vi "LOERN_GetTerms.vi"(0 "XRef":T12, 1 "State In":T10={"Inputs"=1, "SelectedIndex"=1, "ClassInfo"=[]}) -> (14 "Terms":T2, 15 "Fatal Error Out":T1)   [LabVIEW 2016, in "LV Object Event Registration Node.xnode"]
uses:
  LV Object Event Registration Node.xnode
  <vilib>/XNodeSupport/XNodeXNodeRef.ctl
  LOERN_State.ctl
  LOERN_ClassInfo.ctl
  <vilib>/XNodeSupport/XNodeTerm4Array.ctl
  <vilib>/XNodeSupport/XNodeTerm4.ctl
  <vilib>/XNodeSupport/XNodeString.ctl
  <vilib>/XNodeSupport/XNodeVariant.ctl
  <vilib>/XNodeSupport/XNodeRect32.ctl
  <vilib>/XNodeSupport/XNodeInt.ctl
  <vilib>/XNodeSupport/XNodeBool.ctl
  <vilib>/XNodeSupport/XNodeTermDirection.ctl
  <vilib>/XNodeSupport/XNodeErrorCluster.ctl
  <vilib>/XNodeSupport/NI_XNodeSupport.lvlib
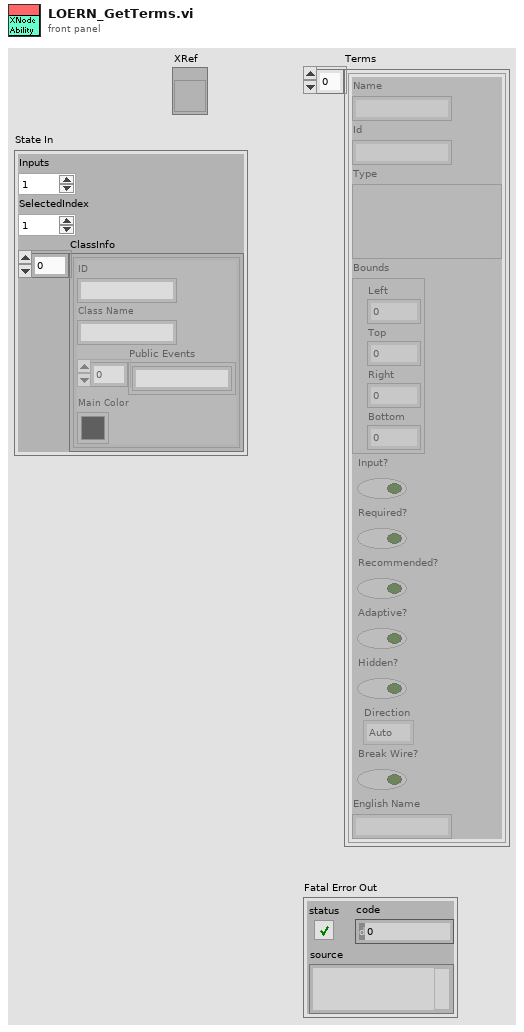
[diagram p1: front panel]
types:
  T1 = typedef "NI_XNodeSupport.lvlib/XNodeErrorCluster.ctl" = errorcluster
  T2 = typedef "NI_XNodeSupport.lvlib/XNodeTerm4Array.ctl" = T3[]
  T3 = typedef "NI_XNodeSupport.lvlib/XNodeTerm4.ctl" = cluster{"Name":T4, "Id":T4, "Type":T5, "Bounds":T6, "Input?":T8, "Required?":T8, "Recommended?":T8, "Adaptive?":T8, "Hidden?":T8, "Direction":T9, "Break Wire?":T8, "English Name":T4}
  T4 = typedef "NI_XNodeSupport.lvlib/XNodeString.ctl" = string
  T5 = typedef "NI_XNodeSupport.lvlib/XNodeVariant.ctl" = variant
  T6 = typedef "NI_XNodeSupport.lvlib/XNodeRect32.ctl" = cluster{"Left":T7, "Top":T7, "Right":T7, "Bottom":T7}
  T7 = typedef "NI_XNodeSupport.lvlib/XNodeInt.ctl" = i32
  T8 = typedef "NI_XNodeSupport.lvlib/XNodeBool.ctl" = bool
  T9 = typedef "NI_XNodeSupport.lvlib/XNodeTermDirection.ctl" = enum32{"Auto", "Up", "Down", "Left", "Right", "Center"}
  T10 = typedef "LV Object Event Registration Node.xnode/LOERN_State.ctl" = cluster{"Inputs":u16, "SelectedIndex":i16, "ClassInfo":T11[]}
  T11 = typedef "LV Object Event Registration Node.xnode/LOERN_ClassInfo.ctl" = cluster{"ID":string, "Class Name":string, "Public Events":string[], "Main Color":u32}
  T12 = typedef "NI_XNodeSupport.lvlib/XNodeXNodeRef.ctl" = refnum<vi>
  T13 = typedef "NI_XNodeSupport.lvlib/XNodeBounds.ctl" = cluster{"Width":T7, "Height":T7}
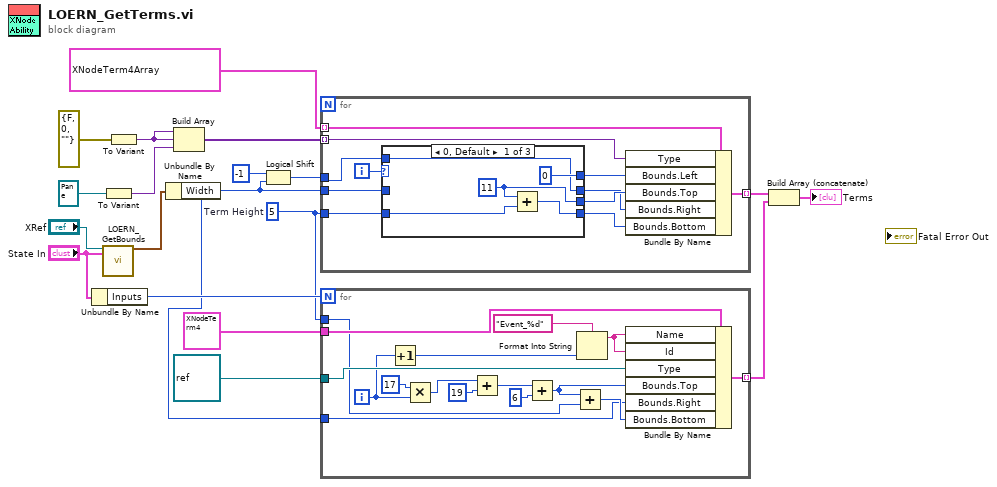
[diagram p0: block diagram]
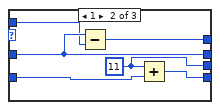
[diagram p2: hidden frame]
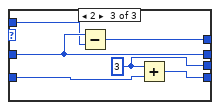
[diagram p3: hidden frame]
diagram:
  w4 = 5  # Term Height
  n1 = Unbundle By Name("State In") -> ("Inputs"=w10:u16)
  n2 = call "LOERN_GetBounds.vi"("XRef"="XRef", "State In"="State In") -> ("Bounds"=w12:T13)  [unwired: 16 in, 1 out]
  n3 = To Variant(anything=refnum<event-registration> refnum ("event registration refnum")) -> (Variant=w15:variant)
  n4 = To Variant(anything=errorcluster {"status"=FALSE, "code"=0, "source"=""} ("error in (no error)")) -> (Variant=w17:variant)
  n5 = Unbundle By Name(w12) -> ("Width"=w3:T7)
  n6 = Build Array(w17, w17, w15) -> (w14:variant[])
  n7 = Logical Shift(y=i16 -1, x=w3) -> (x << y=w1:T7)
  n8 = for {
    tunnel: T2 [{"Name"="Error_In", "Id"="error in", "Type"=variant, "Bounds"={"Left"=0, "Top"=0, "Right"=0, "Bottom"=0}, "Input?"=TRUE, "Required?"=FALSE, "Recommended?"=FALSE, "Adaptive?"=FALSE, "Hidden?"=FALSE, "Direction"=enum."Auto", "Break Wire?"=FALSE, "English Name"=""}, {"Name"="Error_Out", "Id"="error out", "Type"=variant, "Bounds"={"Left"=0, "Top"=0, "Right"=0, "Bottom"=0}, "Input?"=FALSE, "Required?"=FALSE, "Recommended?"=TRUE, "Adaptive?"=FALSE, "Hidden?"=FALSE, "Direction"=enum."Auto", "Break Wire?"=FALSE, "English Name"=""}, {"Name"="Obj_Event_Reg_Ref", "Id"="Object Event Registration Refnum", "Type"=variant, "Bounds"={"Left"=0, "Top"=0, "Right"=0, "Bottom"=0}, "Input?"=FALSE, "Required?"=FALSE, "Recommended?"=TRUE, "Adaptive?"=TRUE, "Hidden?"=FALSE, "Direction"=enum."Auto", "Break Wire?"=FALSE, "English Name"=""}] ("Terms") -> [w30] mode=indexing
    tunnel: w14 -> [w29] mode=indexing
    tunnel: [w28] -> w7 mode=indexing
    tunnel: w3 -> [w22]
    tunnel: w4 -> [w21]
    tunnel: w1 -> [w20]
    i -> [w27]
    n9 = case shown="0, Default" w27 {
      tunnel: [T7 0 ("Bounds.Left") w40 w46] -> w26
      tunnel: [w34 w39 w45] -> w25
      tunnel: [w31 w41 w47] -> w24
      tunnel: [w32 w37 w43] -> w23
      tunnel: w22 -> [_ w41 w47]
      tunnel: w21 -> [w33 w38 w44]
      tunnel: w20 -> [w31 w36 w42]
      frame 0, Default {
        w34 = T7 11 ("Bounds.Left")
        n10 = Add(x=w34, y=w33) -> (x+y=w32:T7)
      }
      frame 1 {
        w39 = T7 11 ("Bounds.Left")
        n11 = Subtract(x=w41, y=w36) -> (x-y=w40:T7)
        n12 = Add(x=w39, y=w38) -> (x+y=w37:T7)
      }
      frame 2 {
        w45 = T7 3 ("Bounds.Left")
        n13 = Subtract(x=w47, y=w42) -> (x-y=w46:T7)
        n14 = Add(x=w45, y=w44) -> (x+y=w43:T7)
      }
    }
    n15 = Bundle By Name(cluster=w30, "Type"=w29, "Bounds.Left"=w26, "Bounds.Top"=w25, "Bounds.Right"=w24, "Bounds.Bottom"=w23) -> (w28:T3)
  }
  n16 = for {
    N: w10 -> [_]
    tunnel: T3 {"Name"="Event", "Id"="Event", "Type"=variant, "Bounds"={"Left"=0, "Top"=0, "Right"=4, "Bottom"=0}, "Input?"=TRUE, "Required?"=TRUE, "Recommended?"=FALSE, "Adaptive?"=TRUE, "Hidden?"=FALSE, "Direction"=enum."Auto", "Break Wire?"=FALSE, "English Name"=""} ("Term 4") -> [w63]
    tunnel: refnum<class> refnum ("LabVIEW Object") -> [w59]
    tunnel: [w58] -> w6 mode=indexing
    tunnel: w4 -> [w50]
    tunnel: w3 -> [w48]
    i -> [w56]
    n17 = Increment(x=w56) -> (x+1=w62:i32)
    n18 = Multiply(x=17, y=w56) -> (x*y=w54:i32)
    n19 = Add(x=w54, y=19) -> (x+y=w53:i32)
    n20 = Add(x=w53, y=6) -> (x+y=w51:i32)
    n21 = Add(x=w51, y=w50) -> (x+y=w49:i32)
    n22 = Format Into String(format string="Event_%d", w62) -> (resulting string=w60:string)  [unwired: 2 in, 1 out]
    n23 = Bundle By Name(cluster=w63, "Name"=w60, "Id"=w60, "Type"=w59, "Bounds.Top"=w51, "Bounds.Right"=w48, "Bounds.Bottom"=w49) -> (w58:T3)
  }
  n24 = Build Array (concatenate)(w7, w6) -> (→"Terms":T3[])
